vi "NT Check Errors.vi"(8 "error in (no error)":errorcluster, 9 "success":u32=1, 10 "pubSubHandle":u32, 11 "topicHandle":u32) -> (0 "error out":errorcluster)   [LabVIEW 2025]
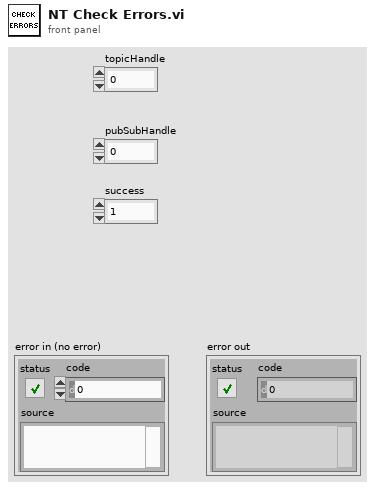
[diagram p1: front panel]
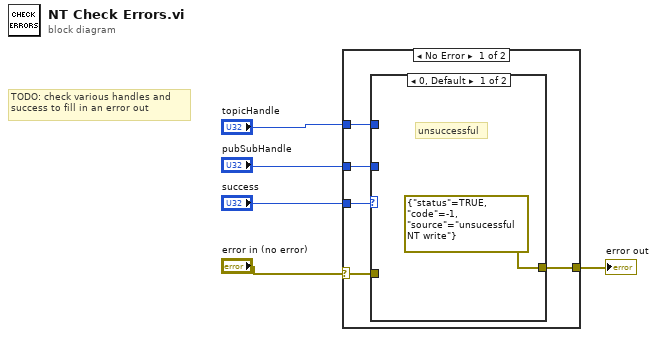
[diagram p0: block diagram]
diagram:
  # "TODO: check various handles and\nsuccess to fill in an error out"
  n1 = case shown="No Error" "error in (no error)" {
    selector: "error in (no error)" -> [w6 w13]
    tunnel: "topicHandle" -> [w10 _]
    tunnel: "pubSubHandle" -> [w9 _]
    tunnel: [w8 w13] -> w3
    tunnel: "success" -> [w7 _]
    frame No Error {
      n2 = case shown="0, Default" w7 {
        tunnel: w6 -> [_ w12]
        tunnel: [errorcluster {"status"=TRUE, "code"=-1, "source"="unsucessful NT write"} ("error IO") w12] -> w8
        tunnel: w9 -> [_ _]
        tunnel: w10 -> [_ _]
        frame 0, Default {
          # "unsuccessful"
        }
        frame 1 {
        }
      }
    }
    frame Error {
    }
  }
  "error out" <- w3
